vi "copy file from another location.vi"() -> ()   [LabVIEW 2023, in "EXIF Modifier.lvlib"]
uses:
  EXIF Modifier.lvlib
panel:
  out "Array":string[](array[string])
  out "Numeric":i32
  in  "Folder Path":path
  out "All Files in Dir":path[](array[path])
  out "Number of Files":i32
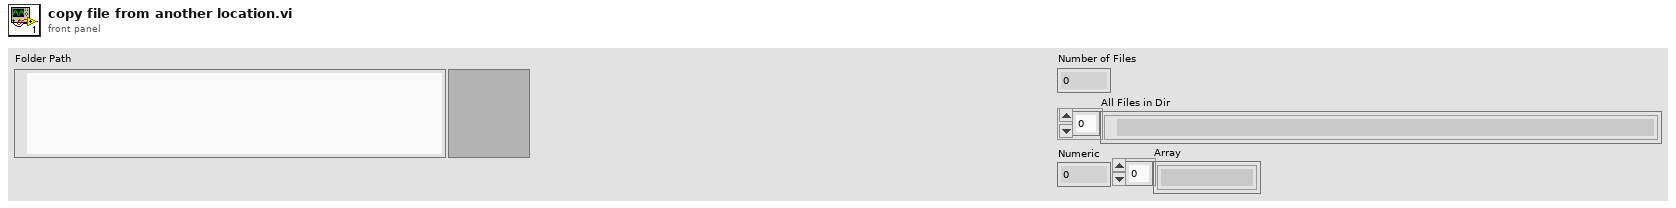
[diagram p1: front panel]
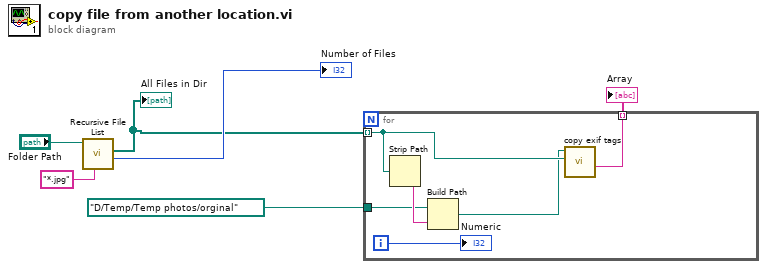
[diagram p0: block diagram]
diagram:
  n1 = call <vilib>:"Recursive File List.vi"("pattern"="*.jpg", "Folder Path"="Folder Path") -> ("Number of Files"=→"Number of Files":i32, "All Files in Dir"=w3:path[])  [unwired: 5 in, 3 out]
  "All Files in Dir" <- w3
  n2 = for {
    tunnel: w3 -> [w12] mode=indexing
    tunnel: path "D:/Temp/Temp photos/orginal" ("base path") -> [w10]
    tunnel: [w7] -> w1 mode=indexing
    i -> [w8]
    n3 = Strip Path(path=w12) -> (name=w11:string)  [unwired: 1 out]
    n4 = Build Path(base path=w10, name or relative path=w11) -> (appended path=w9:path)
    n5 = call "copy exif tags.vi"("destination"=w12, "source"=w9) -> ("standard error"=w7:string)  [unwired: 8 in, 1 out]
    "Numeric" <- w8
  }
  "Array" <- w1
